vi "CheckLockLid.vi"(8 "error in (no error)":errorcluster) -> (0 "error out":errorcluster)   [LabVIEW 2018, in "S4.lvclass"]
uses:
  S4.lvclass
  Public Controls/ReportHeader.ctl
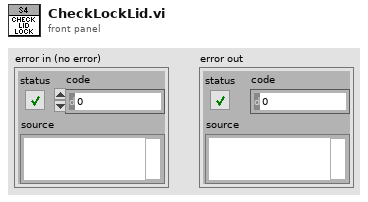
[diagram p1: front panel]
types:
  T1 = typedef "S4.lvclass/ReportHeader.ctl" = string
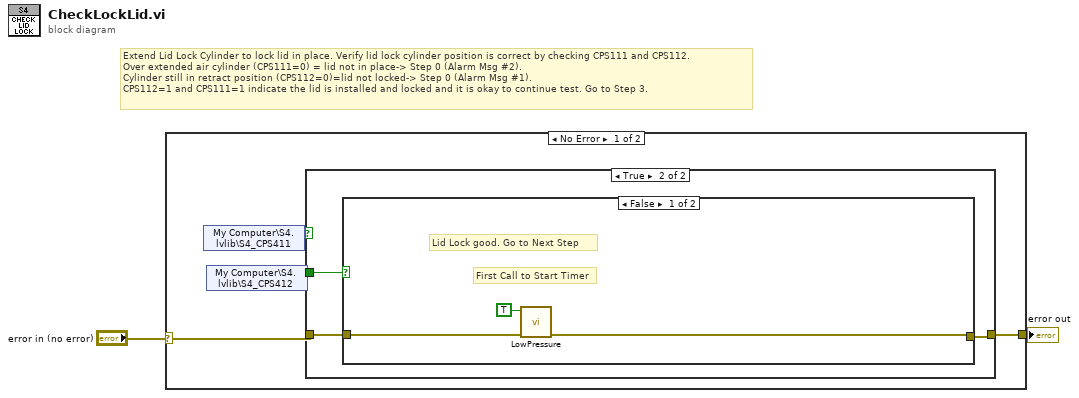
[diagram p0: block diagram]
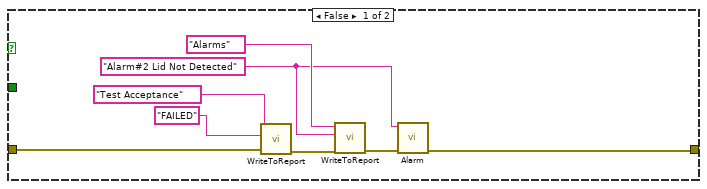
[diagram p2: hidden frame]
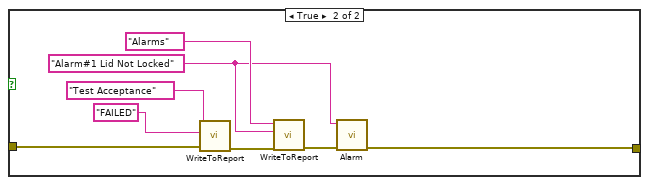
[diagram p3: hidden frame]
diagram:
  # "Extend Lid Lock Cylinder to lock lid in place. Verify lid lock cylinder position is correct by checking CPS111 and CPS112. \nOver extended air cylinder (CPS111=0) = lid not in place-> Step 0 (Alarm Msg #2). \nCylinder still in retract position (CPS112=0)=lid not locked-> Step 0 (Alarm Msg #1). \nCPS112=1 and CPS111=1 indicate the lid is installed and locked and it is okay to continue test. Go to Step 3."
  n1 = case shown="No Error" "error in (no error)" {
    selector: "error in (no error)" -> [w6 w29]
    tunnel: [w5 w29] -> w2
    frame No Error {
      n2 = shared-variable "My Computer\\S4.lvlib\\S4_CPS411"() -> (w4:bool)  [unwired: 1 in, 1 out]
      n3 = shared-variable "My Computer\\S4.lvlib\\S4_CPS412"() -> (w3:bool)  [unwired: 1 in, 1 out]
      n4 = case shown="True" w4 {
        tunnel: w6 -> [w11 w16]
        tunnel: [w10 w15] -> w5
        tunnel: w3 -> [_ w17]
        frame False {
          w7 = "Alarm#2 Lid Not Detected" ("Value")
          n5 = call "WriteToReport.vi"("error in"=w11, "Value"="FAILED", "Header"=T1 "Test Acceptance") -> ("error out"=w14:errorcluster)  [unwired: 8 in]
          n6 = call "WriteToReport.vi"("error in"=w14, "Value"=w7, "Header"="Alarms") -> ("error out"=w12:errorcluster)  [unwired: 8 in]
          n7 = call "Alarm.vi"("error in"=w12, "Alarm"=w7) -> ("error out"=w10:errorcluster)  [unwired: 9 in]
        }
        frame True {
          n8 = case shown="False" w17 {
            tunnel: w16 -> [w20 w28]
            tunnel: [w19 w24] -> w15
            frame False {
              # "First Call to Start Timer"
              # "Lid Lock good. Go to Next Step"
              n9 = call "LowPressure.vi"("error in"=w20, "FirstCall(F)"=TRUE) -> ("error out"=w19:errorcluster)  [unwired: 9 in]
            }
            frame True {
              w22 = "Alarm#1 Lid Not Locked" ("Value")
              n10 = call "WriteToReport.vi"("error in"=w28, "Value"="FAILED", "Header"=T1 "Test Acceptance") -> ("error out"=w27:errorcluster)  [unwired: 8 in]
              n11 = call "WriteToReport.vi"("error in"=w27, "Value"=w22, "Header"="Alarms") -> ("error out"=w25:errorcluster)  [unwired: 8 in]
              n12 = call "Alarm.vi"("error in"=w25, "Alarm"=w22) -> ("error out"=w24:errorcluster)  [unwired: 9 in]
            }
          }
        }
      }
    }
    frame Error {
    }
  }
  "error out" <- w2
